vi "Delivery - broadcast.vi"(8 "error in (no error)":errorcluster) -> (0 "error out":errorcluster)   [LabVIEW 2026, in "Tests.lvlib"]
doc: "Integration test. Verifies that a single Log call fans out to every registered appender: registers three queue-mode relay appenders, logs one Info message, and asserts each appender's queue receives exactly one Statement with identical payload. Every gate except fan-out is held open (global threshold at floor, permissive filters, unbounded queues), so a missing element can only be a fan-out defect."
uses:
  Tests.lvlib
  src/TypeDefs/Severity.ctl
  <vilib>/addons/_JKI Toolkits/Caraya/classes/Assert/Assert False.vi
  <vilib>/addons/_JKI Toolkits/Caraya/classes/Assert/Assert Equal Value_Variant.vi
  <vilib>/addons/_JKI Toolkits/Caraya/classes/Assert/Assert True.vi
  <vilib>/addons/_JKI Toolkits/Caraya/classes/Test/Test.lvclass
  src/Lumberjack.lvlib
  src/Public/Logger.lvclass/Logger.lvclass
  <vilib>/addons/_JKI Toolkits/Caraya/classes/Assert/Assert.lvclass
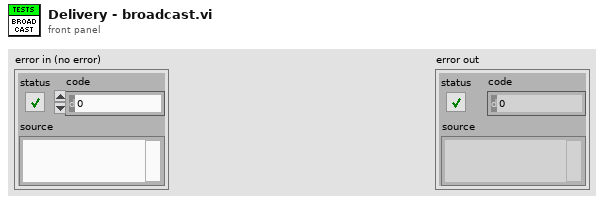
[diagram p1: front panel]
types:
  T1 = typedef "Lumberjack.lvlib/Severity.ctl" = enum16{"OFF", "FATAL", "ERROR", "WARN", "INFO", "DEBUG", "TRACE", "ALL"}
  T2 = typedef "Lumberjack.lvlib/Statement.ctl" = cluster{"timestamp":timestamp, "level":T1, "sourceTag":string, "originVI":string, "message":string}
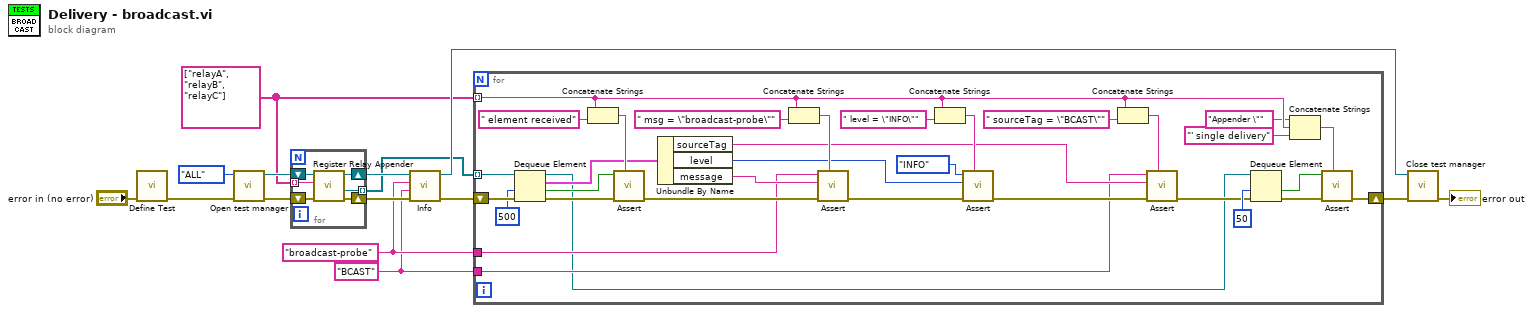
[diagram p0: block diagram]
diagram:
  w2 = "BCAST" ("sourceTag")
  w4 = string[] ["relayA", "relayB", "relayC"]
  w3 = "broadcast-probe" ("message")
  n1 = call <vilib>:"Define Test.vi"("error in (no error)"="error in (no error)") -> ("error out"=w14:errorcluster)  [unwired: 9 in, 1 out]
  n2 = call "Open test manager.vi"("error in (no error)"=w14, "globalThreshold"=Severity."ALL") -> ("error out"=w8:errorcluster, "Logger out"=w9:refnum<class "Logger.lvclass">)  [unwired: 8 in]
  n3 = for {
    shift-right: [w19] -> w7
    shift-left: w9 -> [w21]
    shift-right: [w18] -> w6
    shift-left: w8 -> [w20]
    tunnel: w4 -> [w17] mode=indexing
    tunnel: [w16] -> w5 mode=indexing
    n4 = call "Register Relay Appender.vi"("error in (no error)"=w20, "id in"=w17, "Logger in"=w21) -> ("error out"=w18:errorcluster, "relayQueue"=w16:refnum<queue>, "Logger out"=w19:refnum<class "Logger.lvclass">)  [unwired: 5 in, 1 out]
  }
  n5 = call "Info.vi"("error in (no error)"=w6, "sourceTag"=w2, "message"=w3, "Logger in"=w7) -> ("error out"=w12:errorcluster, "Logger out"=w10:refnum<class "Logger.lvclass">)  [unwired: 6 in]
  n6 = for {
    shift-right: [w26] -> w1
    shift-left: w12 -> [w54]
    tunnel: w5 -> [w52] mode=indexing
    tunnel: w4 -> [w24] mode=indexing
    tunnel: w3 -> [w30]
    tunnel: w2 -> [w31]
    n7 = Dequeue Element(queue=w52, timeout in ms (-1)=500, error in (no error)=w54) -> (queue out=w28:refnum<queue>, element=w46:T2, timed out?=w49:bool, error out=w51:errorcluster)
    n8 = Concatenate Strings(w24, " element received" ("Label")) -> (w47:string)
    n9 = call-poly <vilib>:"Assert.vi"("Label"=w47, "error in (no error)"=w51, "False?"=w49) -> ("error out"=w50:errorcluster)  [unwired: 7 in, 1 out]
    n10 = Unbundle By Name(w46) -> ("sourceTag"=w32:string, "level"=w39:T1, "message"=w43:string)
    n11 = Concatenate Strings(w24, " msg = \"broadcast-probe\"" ("Label")) -> (w41:string)
    n12 = call-poly <vilib>:"Assert.vi"("Label"=w41, "error in (no error)"=w50, "Actual"=w43, "Expected"=w30) -> ("error out"=w45:errorcluster)  [unwired: 6 in, 1 out]
    n13 = Concatenate Strings(w24, " level = \"INFO\"" ("Label")) -> (w37:string)
    n14 = call-poly <vilib>:"Assert.vi"("Label"=w37, "error in (no error)"=w45, "Actual"=w39, "Expected"=Severity."INFO" ("level")) -> ("error out"=w44:errorcluster)  [unwired: 6 in, 1 out]
    n15 = Concatenate Strings(w24, " sourceTag = \"BCAST\"" ("Label")) -> (w29:string)
    n16 = call-poly <vilib>:"Assert.vi"("Label"=w29, "error in (no error)"=w44, "Actual"=w32, "Expected"=w31) -> ("error out"=w34:errorcluster)  [unwired: 6 in, 1 out]
    n17 = Dequeue Element(queue=w28, timeout in ms (-1)=50, error in (no error)=w34) -> (timed out?=w27:bool, error out=w33:errorcluster)  [unwired: 2 out]
    n18 = Concatenate Strings("Appender \"" ("string"), w24, "' single delivery" ("Label")) -> (w22:string)
    n19 = call-poly <vilib>:"Assert.vi"("Label"=w22, "error in (no error)"=w33, "True?"=w27) -> ("error out"=w26:errorcluster)  [unwired: 7 in, 1 out]
  }
  n20 = call "Close test manager.vi"("error in (no error)"=w1, "Logger in"=w10) -> ("error out"=→"error out":errorcluster)  [unwired: 9 in]
